vi "UMB_scaleGoodness.vi"(1 "goodness":dbl[](array[numeric])) -> (0 "scaled goodness":dbl[](array[numeric]))   [LabVIEW 2012]
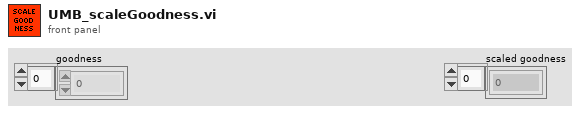
[diagram p1: front panel]
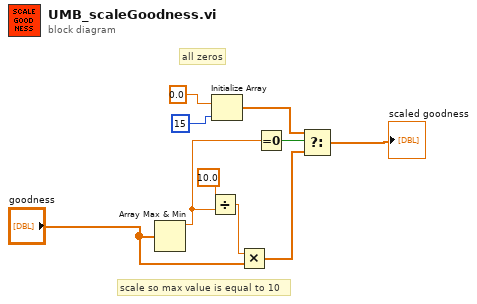
[diagram p0: block diagram]
diagram:
  # "all zeros"
  # "scale so max value is equal to 10"
  n1 = Array Max & Min(array="goodness") -> (max value=w5:dbl)  [unwired: 3 out]
  n2 = Divide(x=10.0, y=w5) -> (x/y=w9:dbl)
  n3 = Initialize Array(0.0 ("element"), 15 ("dimension size")) -> (w3:dbl[])
  n4 = Multiply(x=w9, y="goodness") -> (x*y=w2:dbl[])
  n5 = Equal To 0?(x=w5) -> (x = 0?=w4:bool)
  n6 = Select(t=w3, s=w4, f=w2) -> (s? t:f=→"scaled goodness":dbl[])
